vi "Write Name.vi"(8 "error in (no error)":errorcluster, 10 "Name":string="Name", 11 "Sensor in":refnum<class "Sensor.lvclass">) -> (0 "error out":errorcluster, 3 "Sensor out":refnum<class "Sensor.lvclass">)   [LabVIEW 2012, in "Sensor Definition.lvlib" / "Sensor.lvclass"]
uses:
  Sensor.lvclass
  Sensor.lvclass/Sensor.ctl
  SensorInfo.lvclass/SensorInfo.ctl
  SensorInfo.lvclass
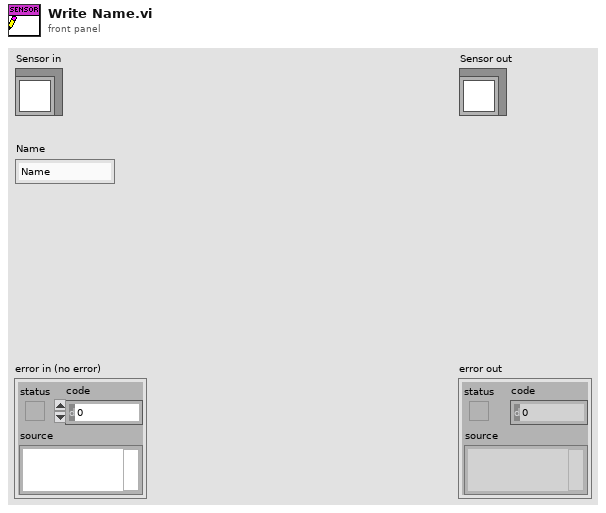
[diagram p1: front panel]
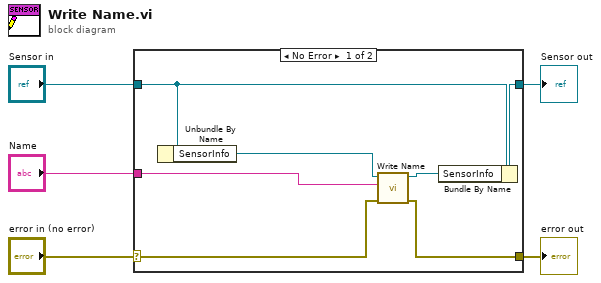
[diagram p0: block diagram]
diagram:
  n1 = case shown="No Error" "error in (no error)" {
    selector: "error in (no error)" -> [w7 w13]
    tunnel: [w6 w13] -> w4
    tunnel: [w12 w14] -> w2
    tunnel: "Sensor in" -> [w11 w14]
    tunnel: "Name" -> [w9 _]
    frame No Error {
      n2 = Unbundle By Name(w11) -> ("SensorInfo"=w10:refnum<class "SensorInfo.lvclass">)
      n3 = call "Write Name.vi"("error in (no error)"=w7, "Name"=w9, "SensorInfo in"=w10) -> ("error out"=w6:errorcluster, "SensorInfo out"=w8:refnum<class "SensorInfo.lvclass">)  [unwired: 7 in]
      n4 = Bundle By Name(cluster=w11, "SensorInfo"=w8) -> (w12:refnum<class "Sensor.lvclass">)
    }
    frame Error {
    }
  }
  "error out" <- w4
  "Sensor out" <- w2
